vi "Final_tranning.vi"() -> ()   [LabVIEW 2017]
panel:
  in  "TriggerRate":u8(ring)=5 items=["125Hz", "250Hz", "500Hz", "1000Hz", "10000Hz", "20000Hz", "50000Hz"]
  in  "String":string
  in  "Train":bool
  in  "address":string="192.168.10.35"
  in  "error in (no error)":errorcluster
  out "error out":errorcluster
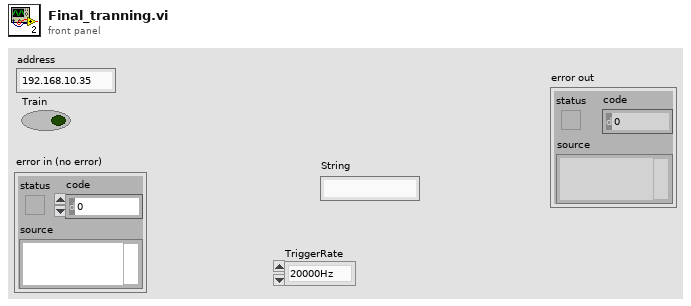
[diagram p1: front panel]
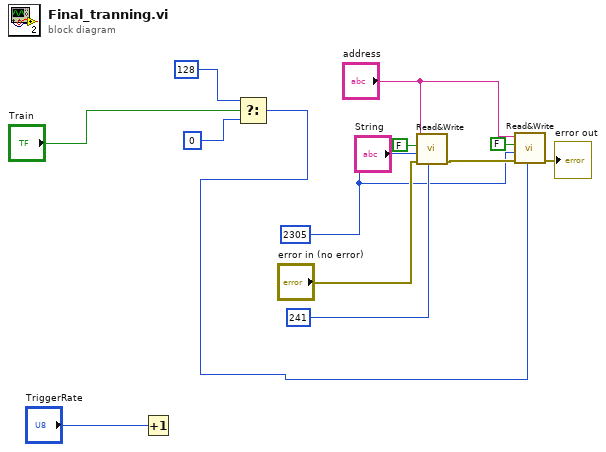
[diagram p0: block diagram]
diagram:
  w6 = u32 2305 ("Address")
  n1 = Increment(x="TriggerRate") -> ()  [unwired: 1 out]
  n2 = Select(t=u8 128 ("In 3"), s="Train", f=u8 0 ("In 3")) -> (s? t:f=w1:u8)
  n3 = call "Read&Write.vi"("In"=u8 241, "error in (no error)"="error in (no error)", "Address"=w6, "Read (TRUE)"=FALSE, "address"="address") -> ("error out"=w13:errorcluster)  [unwired: 5 in, 1 out]
  n4 = call "Read&Write.vi"("In"=w1, "error in (no error)"=w13, "Address"=w6, "Read (TRUE)"=FALSE, "address"="address") -> ("error out"=→"error out":errorcluster)  [unwired: 5 in, 1 out]
